vi "Set CompactSubObj.vi"(8 "error in":errorcluster, 10 "Value":refnum<class "Value.lvclass">, 11 "Object Type in":refnum<class "Object Type Base.lvclass">) -> (0 "error out":errorcluster, 3 "Object Type out":refnum<class "Object Type Base.lvclass">)   [LabVIEW 2024, in "Electronic Datasheet.lvlib" / "Object Type Base.lvclass"]
uses:
  Object Type Base.lvclass
  Value/Value.lvclass
  Object Type Base.lvclass/Object Type Base.ctl
  Electronic Datasheet.lvlib
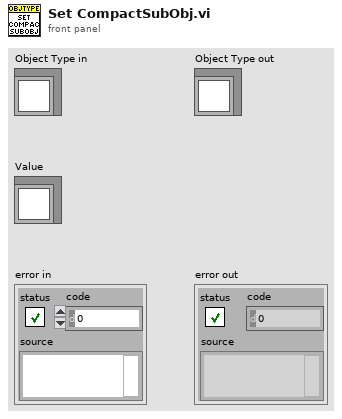
[diagram p1: front panel]
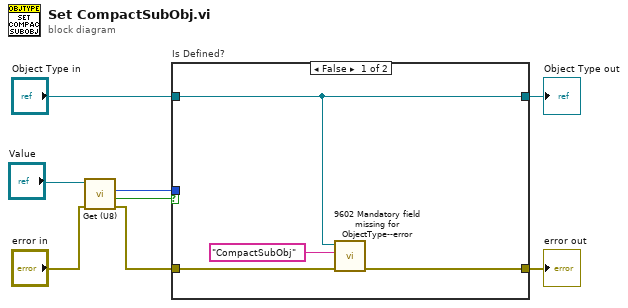
[diagram p0: block diagram]
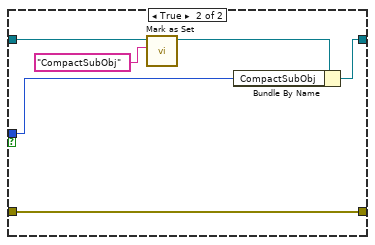
[diagram p2: hidden frame]
diagram:
  n1 = call "Get (U8).vi"("error in"="error in", "Value in"="Value") -> ("error out"=w2:errorcluster, "Defined?"=w4:bool, "Value"=w3:u8)  [unwired: 6 in, 1 out]
  n2 = case "Is Defined?" shown="False" w4 {
    tunnel: "Object Type in" -> [w10 w18]
    tunnel: [w10 w14] -> w7
    tunnel: w3 -> [_ w13]
    tunnel: w2 -> [w12 w16]
    tunnel: [w11 w16] -> w1
    frame False {
      n3 = call "9602 Mandatory field missing for ObjectType--error.vi"("error in"=w12, "Field Name"="CompactSubObj", "Object Type Base"=w10) -> ("error out"=w11:errorcluster)  [unwired: 8 in]
    }
    frame True {
      n4 = call "Mark as Set.vi"("Field name"="CompactSubObj", "Object Type in"=w18) -> ("Object Type out"=w15:refnum<class "Object Type Base.lvclass">)  [unwired: 9 in]
      n5 = Bundle By Name(cluster=w15, "CompactSubObj"=w13) -> (w14:refnum<class "Object Type Base.lvclass">)
    }
  }
  "error out" <- w1
  "Object Type out" <- w7
